vi "convert um to ps.vi"(1 "Position (um)":dbl) -> (0 "Delay (ps)":dbl)   [LabVIEW 2019, in "Instrument.Aerotech.lvclass"]
uses:
  Instrument.Aerotech.lvclass
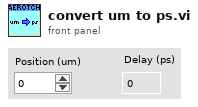
[diagram p1: front panel]
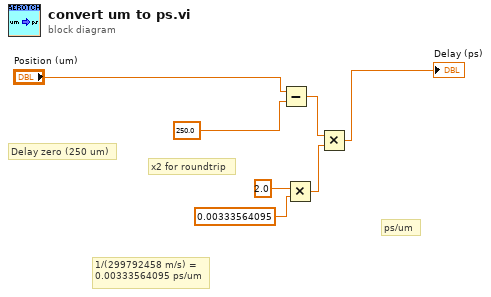
[diagram p0: block diagram]
diagram:
  # "ps/um"
  # "1/(299792458 m/s) = \n0.00333564095 ps/um"
  # "x2 for roundtrip"
  # "Delay zero (250 um)"
  n1 = Subtract(x="Position (um)", y=250.0 ("Time delay zero position (um)")) -> (x-y=w1:dbl)
  n2 = Multiply(x=2.0, y=0.00333564095) -> (x*y=w2:dbl)
  n3 = Multiply(x=w1, y=w2) -> (x*y=→"Delay (ps)":dbl)
